vi "1 V Offset.vi"(1 "Input Data":dbl[][](array[numeric])) -> (0 "Output Data":dbl[][](array[numeric]))   [LabVIEW 2009]
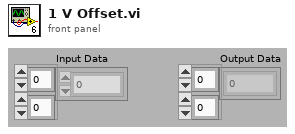
[diagram p1: front panel]
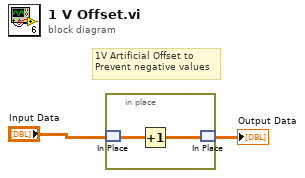
[diagram p0: block diagram]
diagram:
  # "1V Artificial Offset to \nPrevent negative values"
  n1 = in-place {
    n2 = in-place-match #1("Input Data") -> (w4:dbl[][])
    n3 = Increment(x=w4) -> (x+1=w3:dbl[][])
    n4 = in-place-match #1(w3) -> (→"Output Data":dbl[][])
  }
